vi "PID.vi"(8 "error in (no error)":errorcluster, 11 "Sonicator Module State Cluster in":T1={"State"=enum."Idle", "Start Time"=timestamp(0 s since 1904-01-01), "Current Time"=timestamp(0 s since 1904-01-01), "Sonicator Module Config"={"GUID"="", "Drop Coords"={"Horizontal"=0, "Vertical"=0}, "Process Name"="", "User name"="", "Queue Name"="", "Settings"={"Cycle Period"=500.0, "Sonicator Type"="", "SS P100 Settings"={"VISA resource name"="", "Simulated?"=FALSE}, "Setpoint (µm)"=0.0, "Cutoff (W)"=0.0}, "Load Count"=0}, "Output Error"=FALSE, "Log Started"=FALSE, "First Iteration"=FALSE, "Data"={"Sonicator Amp Value"=0.0, "Sonicator Power Value"=0.0, "PID output"=0.0}, "Sonicator On?"=enum."Off"}) -> (0 "error out":errorcluster, 3 "Sonicator Module State Cluster out":T1={"State"=enum."Idle", "Start Time"=timestamp(0 s since 1904-01-01), "Current Time"=timestamp(0 s since 1904-01-01), "Sonicator Module Config"={"GUID"="", "Drop Coords"={"Horizontal"=0, "Vertical"=0}, "Process Name"="", "User name"="", "Queue Name"="", "Settings"={"Cycle Period"=500.0, "Sonicator Type"="", "SS P100 Settings"={"VISA resource name"="", "Simulated?"=FALSE}, "Setpoint (µm)"=0.0, "Cutoff (W)"=0.0}, "Load Count"=0}, "Output Error"=FALSE, "Log Started"=FALSE, "First Iteration"=FALSE, "Data"={"Sonicator Amp Value"=0.0, "Sonicator Power Value"=0.0, "PID output"=0.0}, "Sonicator On?"=enum."Off"})   [LabVIEW 2021, in "Sonicator Module.lvlib" / "Sonicator Module Engine.lvlib"]
uses:
  Sonicator Module Engine.lvlib
  Feed Module/Controls/Sonicator Module State Cluster.ctl
  Pump Module Folder/Measure Instrument/State Enum.ctl
  Feed Module/Controls/Sonicator Module Config Cluster.ctl
  <vilib>/Utility/miscctls.llb/LVPoint32TypeDef.ctl
  Feed Module/Controls/Sonicator Module Settings Cluster.ctl
  Sonic Systems P100/Sonic Systems P100 Settings.ctl
  <vilib>/addons/control/pid/pid.llb/PID Advanced (DBL).vi
  <vilib>/addons/control/pid/NI_PID_pid.lvlib
  Sonic Systems P100/Sonic Systems P100.lvlib
  Sonicator Module.lvlib
  Pump Module Folder/Measure Instrument/Pump Module Engine.lvlib
panel:
  # "Sonicator Settings"
  # "Sonicator Settings"
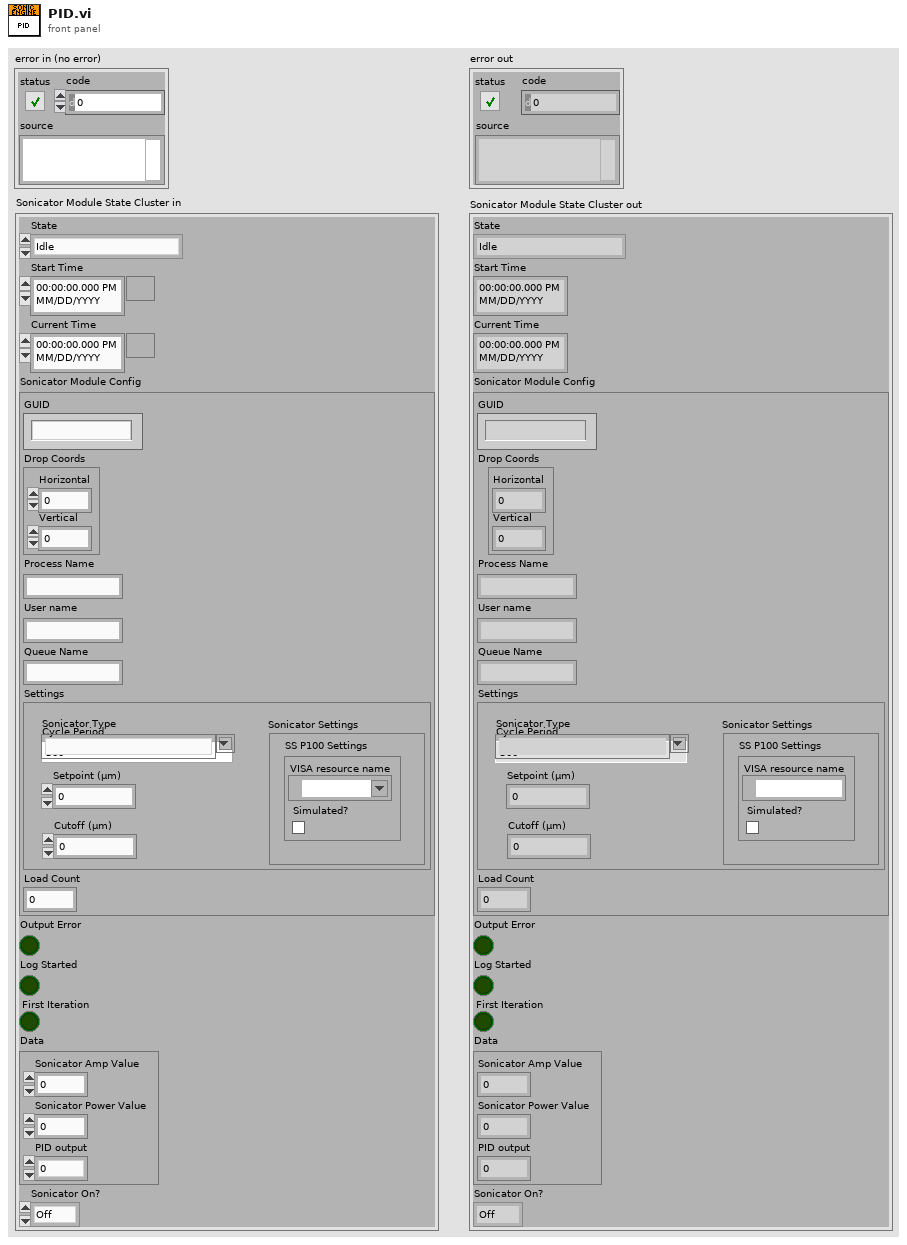
[diagram p1: front panel]
types:
  T1 = typedef "Sonicator Module.lvlib/Sonicator Module State Cluster.ctl" = cluster{"State":T2, "Start Time":timestamp, "Current Time":timestamp, "Sonicator Module Config":T3, "Output Error":bool, "Log Started":bool, "First Iteration":bool, "Data":cluster{"Sonicator Amp Value":dbl, "Sonicator Power Value":dbl, "PID output":dbl}, "Sonicator On?":enum16{"Off", "On", "Not Initialized", "Over Cutoff"}}
  T2 = typedef "Pump Module.lvlib/Pump Module Engine.lvlib/State Enum.ctl" = enum16{"Measuring", "Idle", "Paused"}
  T3 = typedef "Sonicator Module.lvlib/Sonicator Module Config Cluster.ctl" = cluster{"GUID":string, "Drop Coords":T4, "Process Name":string, "User name":string, "Queue Name":string, "Settings":T5, "Load Count":i32}
  T4 = typedef "LVPoint32TypeDef.ctl" = cluster{"Horizontal":i32, "Vertical":i32}
  T5 = typedef "Sonicator Module.lvlib/Sonicator Module Settings Cluster.ctl" = cluster{"Cycle Period":dbl, "Sonicator Type":string, "SS P100 Settings":T6, "Setpoint (µm)":dbl, "Cutoff (W)":dbl}
  T6 = typedef "Sonic Systems P100.lvlib/Sonic Systems P100 Settings.ctl" = cluster{"VISA resource name":refnum<visa-resource-name>, "Simulated?":bool}
  T7 = cluster{"proportional gain (Kc)":dbl, "integral time (Ti, min)":dbl, "derivative time (Td, min)":dbl}
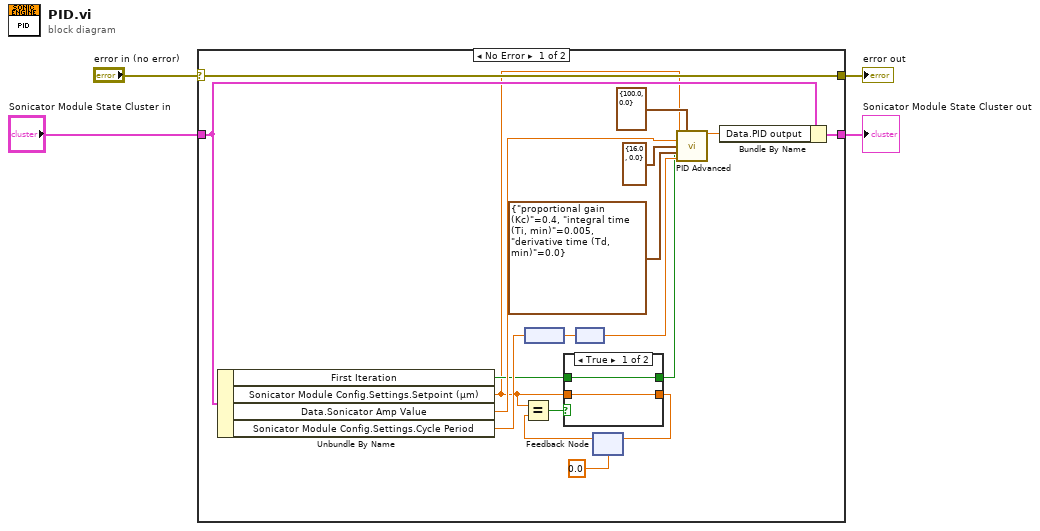
[diagram p0: block diagram]
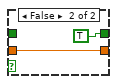
[diagram p2: hidden frame]
diagram:
  n1 = case shown="No Error" "error in (no error)" {
    selector: "error in (no error)" -> [w20 w28]
    tunnel: [w20 w28] -> w3
    tunnel: [w19 w27] -> w1
    tunnel: "Sonicator Module State Cluster in" -> [w13 w27]
    frame No Error {
      n2 = Unbundle By Name(w13) -> ("First Iteration"=w11:bool, "Sonicator Module Config.Settings.Setpoint (µm)"=w7:dbl, "Data.Sonicator Amp Value"=w12:dbl, "Sonicator Module Config.Settings.Cycle Period"=w16:dbl)
      n3 = node(w16) -> (w22:dbl[unit])
      n4 = node(w22) -> (w21:dbl)
      n5 = feedback #1(0.0 ("Setpoint (µm)")) -> (w8:dbl)
      n6 = Equal?(x=w7, y=w8) -> (x = y?=w6:bool)
      n7 = case shown="True" w6 {
        tunnel: w11 -> [w24 _]
        tunnel: [w24 TRUE] -> w10
        tunnel: [w23 w25] -> w9
        tunnel: w7 -> [w23 w25]
        frame True {
        }
        frame False {
        }
      }
      n8 = feedback-in #1(w9) -> ()
      n9 = call-poly <vilib>:"PID Advanced.vi"("setpoint"=w7, "output range"=cluster{"output high":dbl, "output low":dbl} {"output high"=100.0, "output low"=0.0}, "process variable"=w12, "setpoint range"=cluster{"setpoint high":dbl, "setpoint low":dbl} {"setpoint high"=16.0, "setpoint low"=0.0}, "PID gains"=T7 {"proportional gain (Kc)"=0.4, "integral time (Ti, min)"=0.005, "derivative time (Td, min)"=0.0}, "dt (s)"=w21, "reinitialize? (F)"=w10) -> ("output"=w17:dbl)  [unwired: 7 in, 1 out]
      n10 = Bundle By Name(cluster=w13, "Data.PID output"=w17) -> (w19:T1)
    }
    frame Error {
    }
  }
  "error out" <- w3
  "Sonicator Module State Cluster out" <- w1
